vi "Change_More_Generix.vi"(0 "Control_In":refnum<vi>, 5 "Reference_In":refnum<vi>[](array[refnum])) -> (4 "Reference_Out":refnum<vi>[](array[refnum]))   [LabVIEW 2021]
doc: "Used to convert the reference to more generic"
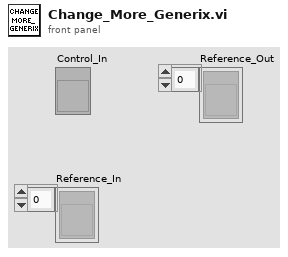
[diagram p1: front panel]
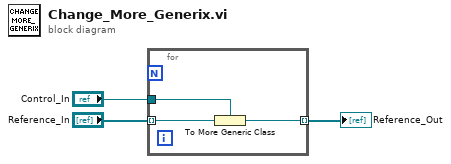
[diagram p0: block diagram]
diagram:
  n1 = for {
    tunnel: "Reference_In" -> [w6] mode=indexing
    tunnel: [w5] -> w2 mode=indexing
    tunnel: "Control_In" -> [w4]
    n2 = To More Generic Class(target class=w4, reference=w6) -> (generic class reference=w5:refnum<vi>)
  }
  "Reference_Out" <- w2
